vi "Test App Get Deeply Nested Process by Qualified Name from Middle.vi"(8 "error in (no error)":errorcluster, 11 "Application Test in":refnum<class "Application Test.lvclass">) -> (0 "error out":errorcluster, 3 "Application Test out":refnum<class "Application Test.lvclass">)   [LabVIEW 2020, in "Application Test.lvclass"]
uses:
  Application Test.lvclass
  C:/Program Files (x86)/National Instruments/LabVIEW 2020/vi.lib/Asteme/LUnit/Test Case.lvclass
  Framework/Process/Process.lvclass
  Framework/Process/Process.lvclass/Process.ctl
  Framework/Application/Application.lvclass/Application.ctl
  <vilib>/Asteme/LUnit/Test Case.lvclass/Test Case.ctl
  <vilib>/Asteme/LUnit/LUnit Assertion Result.lvclass/LUnit Assertion Result.ctl
  Framework/Application/Private/Add Process to Map.vi
  Framework/Application/Private/Start Idle Processes if Running.vi
  Framework/Process/Protected/Messaging/Enqueue Message.vi
  Framework/Process/Public/Lifecycle/Get Lifecycle State.vi
  Framework/Process/Protected/SubVIs/Set Context.vi
  <vilib>/Asteme/LUnit/Palette/Pass.vi
  <vilib>/Asteme/LUnit/Palette/Fail.vi
  <vilib>/Asteme/LUnit/Set Assertion Type.vi
  Framework/Process/Private/SubVIs/Wait for finish.vi
  Framework/Process/Private/SubVIs/Set Lifecycle State.vi
  <vilib>/Utility/error.llb/Clear Errors.vi
  Framework/Process/Public/Lifecycle/Leave Process Loop.vi
  <vilib>/Asteme/LUnit/Add test result.vi
  <vilib>/Asteme/LUnit/LUnit Write Passed.vi
  <vilib>/Asteme/LUnit/LUnit Get Test Case.vi
  <vilib>/Asteme/LUnit/Assertion Result/LUnit Get Test Name.vi
  <vilib>/Asteme/LUnit/LUnit Write Message.vi
  <vilib>/Asteme/LUnit/LUnit Write Description.vi
  <vilib>/Asteme/LUnit/LUnit Write Assertion Type.vi
  <vilib>/Asteme/LUnit/Read Test Case Name.vi
  Framework/Application/Application.lvclass
  C:/Users/anton/Documents/GitHub/Triarc-Framework/source/Framework/Process/Process.lvclass
  <vilib>/Utility/error.llb/Error Cluster From Error Code.vi
  Framework/Application/Private/Update Context for Owned Processes.vi
  <vilib>/Asteme/LUnit/LUnit Assertion Result.lvclass
  <vilib>/Asteme/LUnit/Test Case.lvclass
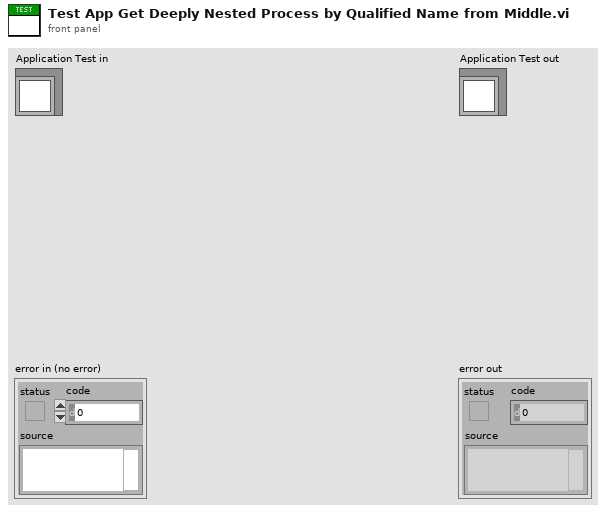
[diagram p1: front panel]
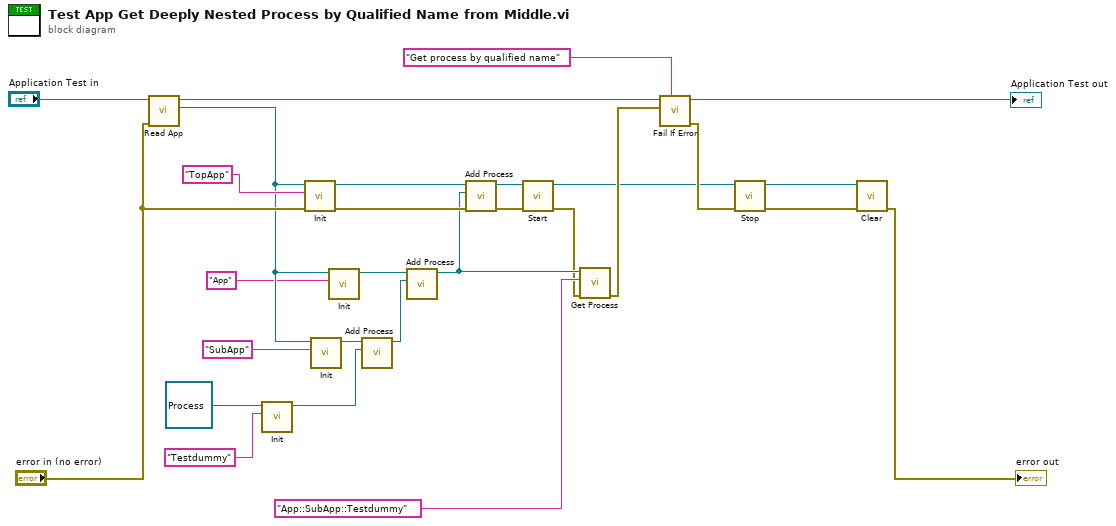
[diagram p0: block diagram]
diagram:
  n1 = call "Read App.vi"("error in (no error)"="error in (no error)", "Application Test In"="Application Test in") -> ("App out"=w11:refnum<class "Application.lvclass">, "Application Test Out"=w28:refnum<class "Application Test.lvclass">)  [unwired: 7 in, 1 out]
  n2 = call-dynamic "Init.vi"("Name"="Testdummy", "Process In"=refnum<class "Process.lvclass"> refnum ("Process.lvclass")) -> ("Process Out"=w12:refnum<class "Process.lvclass">)  [unwired: 8 in, 1 out]
  n3 = call-dynamic "Init.vi"("error in (no error)"="error in (no error)", "Name"="TopApp", "Process In"=w11) -> ("error out"=w26:errorcluster, "Process Out"=w27:refnum<class "Application.lvclass">)  [unwired: 7 in]
  n4 = call-dynamic "Init.vi"("Name"="SubApp", "Process In"=w11) -> ("Process Out"=w13:refnum<class "Application.lvclass">)  [unwired: 8 in, 1 out]
  n5 = call-dynamic "Init.vi"("Name"="App", "Process In"=w11) -> ("Process Out"=w10:refnum<class "Application.lvclass">)  [unwired: 8 in, 1 out]
  n6 = call "Add Process.vi"("Process"=w12, "Rig In"=w13) -> ("Rig Out"=w9:refnum<class "Application.lvclass">)  [unwired: 8 in, 1 out]
  n7 = call "Add Process.vi"("Process"=w9, "Rig In"=w10) -> ("Rig Out"=w7:refnum<class "Application.lvclass">)  [unwired: 8 in, 1 out]
  n8 = call "Add Process.vi"("error in (no error)"=w26, "Process"=w7, "Rig In"=w27) -> ("error out"=w6:errorcluster, "Rig Out"=w2:refnum<class "Application.lvclass">)  [unwired: 7 in]
  n9 = call "Start.vi"("error in (no error)"=w6, "Process In"=w2) -> ("error out"=w3:errorcluster, "Process Out"=w1:refnum<class "Application.lvclass">)  [unwired: 8 in]
  n10 = call "Get Process.vi"("error in (no error)"=w3, "Process Name"="App::SubApp::Testdummy" ("Name"), "Rig In"=w7) -> ("error out"=w5:errorcluster)  [unwired: 6 in, 2 out]
  n11 = call <vilib>:"Fail If Error.vi"("Description"="Get process by qualified name", "Assert error"=w5, "Test Case In"=w28) -> ("error out"=w22:errorcluster, "Test Case Out"=→"Application Test out":refnum<class "Application Test.lvclass">)  [unwired: 7 in]
  n12 = call "Stop.vi"("error in (no error)"=w22, "Process In"=w1) -> ("error out"=w19:errorcluster, "Process Out"=w25:refnum<class "Application.lvclass">)  [unwired: 7 in, 1 out]
  n13 = call-dynamic "Clear.vi"("error in (no error)"=w19, "Application In"=w25) -> ("error out"=→"error out":errorcluster)  [unwired: 9 in]
